vi "综合生物毒性设置窗口.vi"() -> (1 "串口开关状态":bool, 2 "开关":bool, 3 "确定输出":bool)   [LabVIEW 2016, in "综合生物毒性.lvlib"]
uses:
  <vilib>/Plasmionique/MB Master/MB_Master_Serial/MB_Master_Serial.lvclass
  <vilib>/Utility/config.llb/NI_LVConfig.lvlib
  <vilib>/ptbypt/NI_PtbyPt.lvlib
panel:
  in  "设备厂家":string(combo)
  in  "字符串":string
  in  "串口":refnum<visa-resource-name>="COM6"
  in  "确定":bool
  in  "取消":bool
  in  "串口开关":bool
  # "设置综合生物毒性参数"
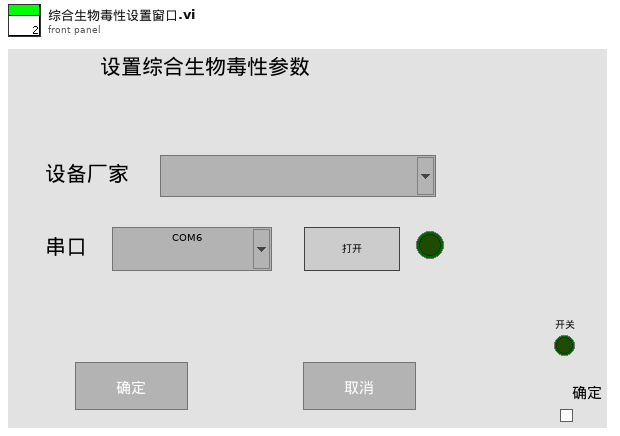
[diagram p1: front panel]
types:
  T1 = enum8{"Enabled", "Disabled", "Disabled and Grayed Out"}
  T2 = cluster{"baud rate (bps)":u32, "stop bits":u16, "parity":u16, "flow control":u16, "timeout":u32, "retries":i32}
  T3 = typedef "NI_LVConfig.lvlib/Config Data RefNum.ctl" = refnum<k1>
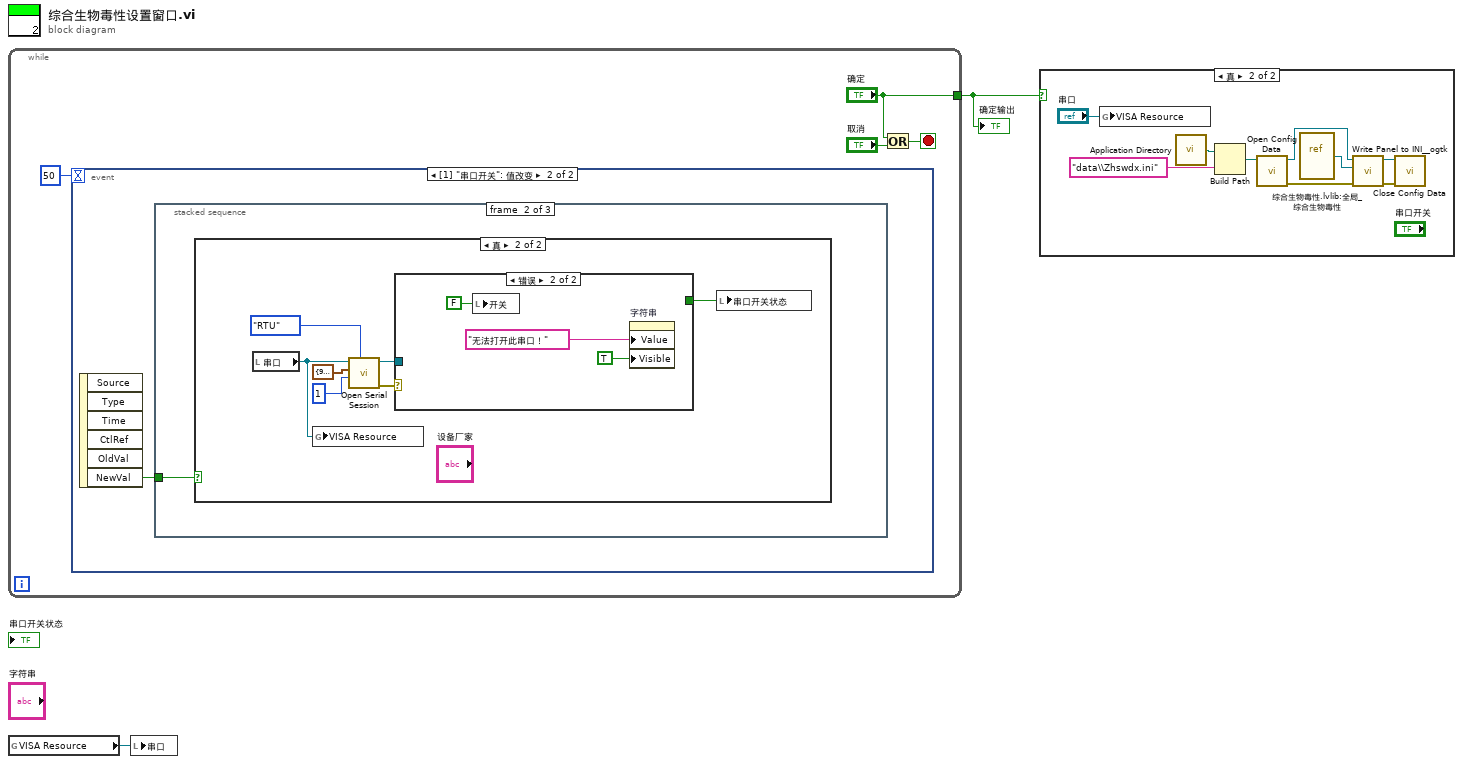
[diagram p0: block diagram]
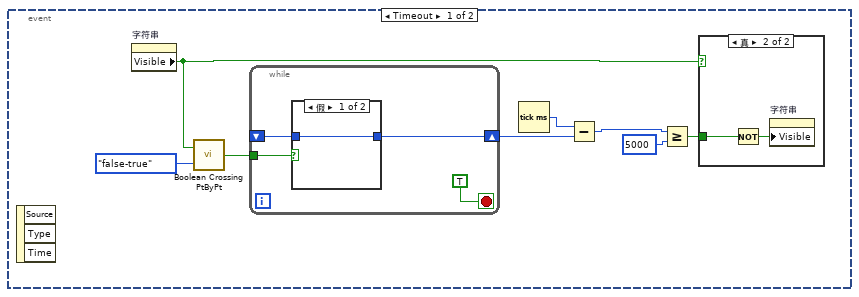
[diagram p3: hidden frame]
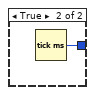
[diagram p5: hidden frame]
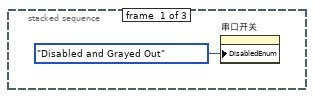
[diagram p6: hidden frame]
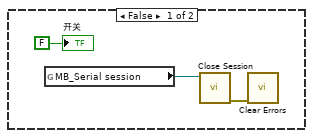
[diagram p7: hidden frame]
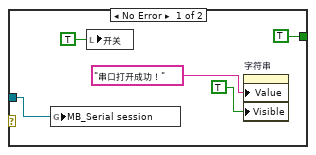
[diagram p8: hidden frame]
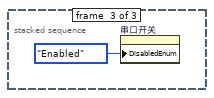
[diagram p9: hidden frame]
diagram:
  n1 = while {
    tunnel: ["确定"] -> w2
    stop <- w4 stop-if-true
    n2 = event shown="[1] \"串口开关\": 值改变" {
      selector: _ -> [_ _]
      dyn-events: _ -> [_ _]
      timeout: 50 -> [_ _]
      event Timeout {
        n3 = event-data() -> ()  [unwired: 1 in, 3 out]
        n4 = property on="字符串" class="Str"() -> ("Visible"=w8:bool)  [unwired: 2 in, 2 out]
        n5 = call <vilib>:"Boolean Crossing PtByPt.vi"("direction"=enum16{"either", "false-true", "true-false"}."false-true", "input"=w8) -> ("crossing"=w13:bool)  [unwired: 1 in]
        n6 = while {
          tunnel: w13 -> [w20]
          shift-right: [w18] -> w11
          shift-left: _ -> [w17]
          stop <- TRUE stop-if-true
          n7 = case shown="假" w20 {
            tunnel: [w21 w22] -> w18
            tunnel: w17 -> [w21 _]
            frame False {
            }
            frame True {
              n8 = Tick Count (ms)() -> (millisecond timer value=w22:u32)
            }
          }
        }
        n9 = Tick Count (ms)() -> (millisecond timer value=w12:u32)
        n10 = Subtract(x=w12, y=w11) -> (x-y=w10:u32)
        n11 = Greater Or Equal?(x=w10, y=u32 5000) -> (x >= y?=w7:bool)
        n12 = case shown="真" w8 {
          tunnel: w7 -> [_ w15]
          frame False {
          }
          frame True {
            n13 = Not(x=w15) -> (.not. x?=w16:bool)
            n14 = property on="字符串" class="Str"("Visible"=w16) -> ()  [unwired: 2 in, 2 out]
          }
        }
      }
      event "串口开关": Value Change {
        n15 = event-data() -> ("NewVal"=w23:bool)  [unwired: 1 in, 5 out]
        n16 = stacked-sequence {
          tunnel: w23 -> [_ w25 _]
          frame #0 {
            n17 = property on="串口开关" class="Bool"("DisabledEnum"=T1."Disabled and Grayed Out" ("禁用")) -> ()  [unwired: 2 in, 2 out]
          }
          frame #1 {
            n18 = case shown="真" w25 {
              frame False {
                n19 = global read "全局_综合生物毒性.vi" "MB_Serial session"() -> (w28:refnum<class "MB_Master_Serial.lvclass">)
                n20 = call-dynamic "Close Session.vi"("MB_Serial session"=w28) -> ("error out"=w27:errorcluster)  [unwired: 10 in]
                n21 = call <vilib>:"Clear Errors.vi"("error in (no error)"=w27) -> ()  [unwired: 5 in, 2 out]
                "开关" <- FALSE ("开关")
              }
              frame True {
                n22 = local read "串口"() -> (w30:refnum<visa-resource-name>)
                n23 = global write "全局_综合生物毒性.vi" "VISA Resource"(w30) -> ()
                n24 = call <vilib>:"Open Serial Session.vi"("Mode (RTU)"=enum16{"RTU", "ASCII"}."RTU", "Slave ID"=u8 1, "Serial Config"=T2 {"baud rate (bps)"=9600, "stop bits"=10, "parity"=0, "flow control"=0, "timeout"=2000, "retries"=1}, "VISA Resource"=w30) -> ("Error out"=w32:errorcluster, "MB_Serial session"=w31:refnum<class "MB_Master_Serial.lvclass">)  [unwired: 6 in]
                n25 = case shown="错误" w32 {
                  tunnel: w31 -> [w40 _]
                  tunnel: [TRUE ("串口开关状态") _] -> w29
                  frame No Error {
                    n26 = global write "全局_综合生物毒性.vi" "MB_Serial session"(w40) -> ()
                    n27 = local write "开关"(TRUE ("开关")) -> ()
                    n28 = property on="字符串" class="Str"("Value"="串口打开成功！" ("字符串"), "Visible"=TRUE ("可见")) -> ()  [unwired: 2 in, 2 out]
                  }
                  frame Error {
                    n29 = local write "开关"(FALSE ("开关")) -> ()
                    n30 = property on="字符串" class="Str"("Value"="无法打开此串口！" ("字符串"), "Visible"=TRUE ("可见")) -> ()  [unwired: 2 in, 2 out]
                  }
                }
                n31 = local write "串口开关状态"(w29) -> ()
              }
            }
          }
          frame #2 {
            n32 = property on="串口开关" class="Bool"("DisabledEnum"=T1."Enabled" ("禁用")) -> ()  [unwired: 2 in, 2 out]
          }
        }
      }
    }
    n33 = Or(x="确定", y="取消") -> (x .or. y?=w4:bool)
  }
  "确定输出" <- w2
  n34 = global read "全局_综合生物毒性.vi" "VISA Resource"() -> (w1:refnum<visa-resource-name>)
  n35 = local write "串口"(w1) -> ()
  n36 = case shown="真" w2 {
    frame False {
    }
    frame True {
      n37 = global write "全局_综合生物毒性.vi" "VISA Resource"("串口") -> ()
      n38 = call <vilib>:"Application Directory.vi"() -> ("Application Directory"=w49:path)
      n39 = Build Path(base path=w49, name or relative path="data\\Zhswdx.ini" ("名称或相对路径")) -> (appended path=w51:path)
      n40 = call <vilib>:"Open Config Data.vi"("configuration file path"=w51) -> ("error out"=w47:errorcluster, "refnum"=w52:T3)  [unwired: 8 in, 1 out]
      n41 = vi-ref "综合生物毒性.lvlib:全局_综合生物毒性.vi"() -> (w46:refnum<vi>)
      n42 = call <userlib>:"Write Panel to INI__ogtk.vi"("error in (no error)"=w47, "VI ref"=w46, "refnum"=w52) -> ("error out"=w48:errorcluster, "refnum out"=w53:T3)  [unwired: 7 in]
      n43 = call <vilib>:"Close Config Data.vi"("error in (no error)"=w48, "refnum"=w53) -> ()  [unwired: 8 in, 2 out]
    }
  }
